vi "Get Discovery Service Address.vi"(8 "error in":errorcluster, 11 "cluster id (\"\")":string) -> (0 "error out":errorcluster, 3 "address":string)   [LabVIEW 2020, in "MeasurementLink Measurement Server.lvlib"]
uses:
  MeasurementLink Measurement Server.lvlib
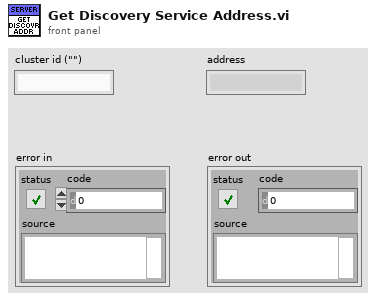
[diagram p1: front panel]
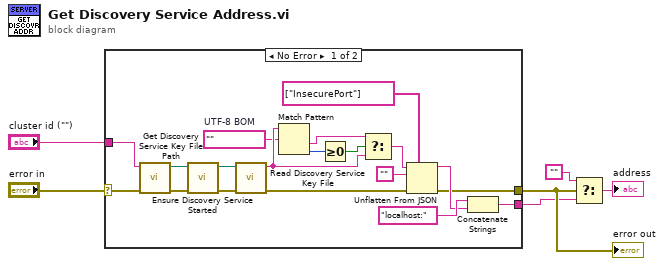
[diagram p0: block diagram]
diagram:
  n1 = case shown="No Error" "error in" {
    selector: "error in" -> [w7 w26]
    tunnel: "cluster id (\"\")" -> [w25 _]
    tunnel: [w13 w26] -> w5
    tunnel: [w12 _] -> w3
    frame No Error {
      w18 = "﻿"  # UTF-8 BOM
      n2 = call "Get Discovery Service Key File Path.vi"("error in (no error)"=w7, "cluster id (\"\")"=w25) -> ("error out"=w11:errorcluster, "key file path"=w9:path)  [unwired: 8 in]
      n3 = call "Ensure Discovery Service Started.vi"("error in (no error)"=w11, "path"=w9) -> ("error out"=w10:errorcluster, "key file path"=w8:path)  [unwired: 8 in]
      n4 = call "Read Discovery Service Key File.vi"("error in (no error)"=w10, "key file path"=w8) -> ("error out"=w16:errorcluster, "key json"=w19:string)  [unwired: 8 in]
      n5 = Match Pattern(string=w19, regular expression=w18) -> (after substring=w22:string, offset past match=w21:i32)  [unwired: 1 in, 2 out]
      n6 = Greater Or Equal To 0?(x=w21) -> (x >= 0?=w23:bool)
      n7 = Select(t=w22, s=w23, f=w19) -> (s? t:f=w24:string)
      n8 = Unflatten From JSON(path=string[] ["InsecurePort"], JSON string=w24, type and defaults="", error in (no error)=w16) -> (value=w14:string, error out=w13:errorcluster)  [unwired: 3 in]
      n9 = Concatenate Strings("localhost:", w14) -> (w12:string)
    }
    frame Error {
    }
  }
  "error out" <- w5
  n10 = Select(t="", s=w5, f=w3) -> (s? t:f=→"address":string)
